vi "Read subDataEvents.vi"(11 "PubSubDataEvent in":refnum<class "PubSubDataEvent.lvclass">) -> (2 "subDataEvents":T1, 3 "PubSubDataEvent out":refnum<class "PubSubDataEvent.lvclass">)   [LabVIEW 2016, in "PubSubDataEvent.lvclass"]
uses:
  PubSubDataEvent.lvclass
  TypedefsDataEvents/SubDataEvents.ctl
  ts_sallv_sedspectrometer/DataTypes/command_disable.ctl
  ts_sallv_sedspectrometer/DataTypes/command_enable.ctl
  ts_sallv_sedspectrometer/DataTypes/command_exitControl.ctl
  ts_sallv_sedspectrometer/DataTypes/command_standby.ctl
  ts_sallv_sedspectrometer/DataTypes/logevent_Heartbeat.ctl
  ts_sallv_sedspectrometer/DataTypes/command_start.ctl
  ts_sallv_sedspectrometer/DataTypes/command_captureSpectImage.ctl
  ts_sallv_sedspectrometer/DataTypes/command_setSpectTempSetpoint.ctl
  ts_sallv_sedspectrometer/DataTypes/command_stopImageCapture.ctl
  PubSubDataEvent.lvclass/PubSubDataEvent.ctl
  TypedefsDataEvents/TypedefsDataEvents.lvlib
  ts_sallv_sedspectrometer/SALLV_sedSpectrometer.lvlib
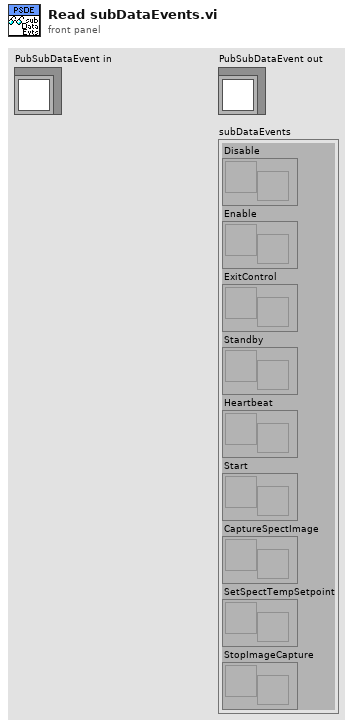
[diagram p1: front panel]
types:
  T1 = typedef "TypedefsDataEvents.lvlib/SubDataEvents.ctl" = cluster{"Disable":refnum<user-event>, "Enable":refnum<user-event>, "ExitControl":refnum<user-event>, "Standby":refnum<user-event>, "Heartbeat":refnum<user-event>, "Start":refnum<user-event>, "CaptureSpectImage":refnum<user-event>, "SetSpectTempSetpoint":refnum<user-event>, "StopImageCapture":refnum<user-event>}
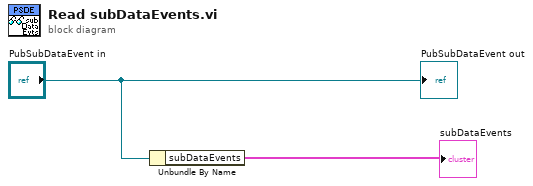
[diagram p0: block diagram]
diagram:
  n1 = Unbundle By Name("PubSubDataEvent in") -> ("subDataEvents"=→"subDataEvents":T1)
  "PubSubDataEvent out" <- "PubSubDataEvent in"
